vi "LHF.DB.Mongo.Client.GetCollectionsName.vi"(0 "LHF.DB.Mongo":refnum<class "LHF.DB.Mongo.lvclass">, 5 "error in (no error)":errorcluster) -> (14 "LHF.DB.Mongo":refnum<class "LHF.DB.Mongo.lvclass">, 15 "Collections":string[](array[string]))   [LabVIEW 2013, in "LHF.DB.Mongo.lvclass"]
uses:
  LHF.DB.Mongo.lvclass
  LHF.DB.Mongo.lvclass/LHF.DB.Mongo.ctl
  C:/Users/schim/Desktop/Projetos/LabVIEW-MongoDB/src/Driver/MongoDB.Driver.dll
  Driver/MongoDB.Driver.dll
  C:/Users/schim/Desktop/Projetos/LabVIEW-MongoDB/src/Driver/MongoDB.Bson.dll
  Driver/MongoDB.Bson.dll
panel:
  out "error out":errorcluster
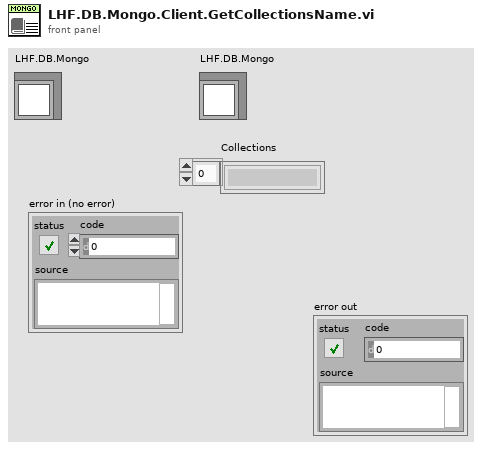
[diagram p1: front panel]
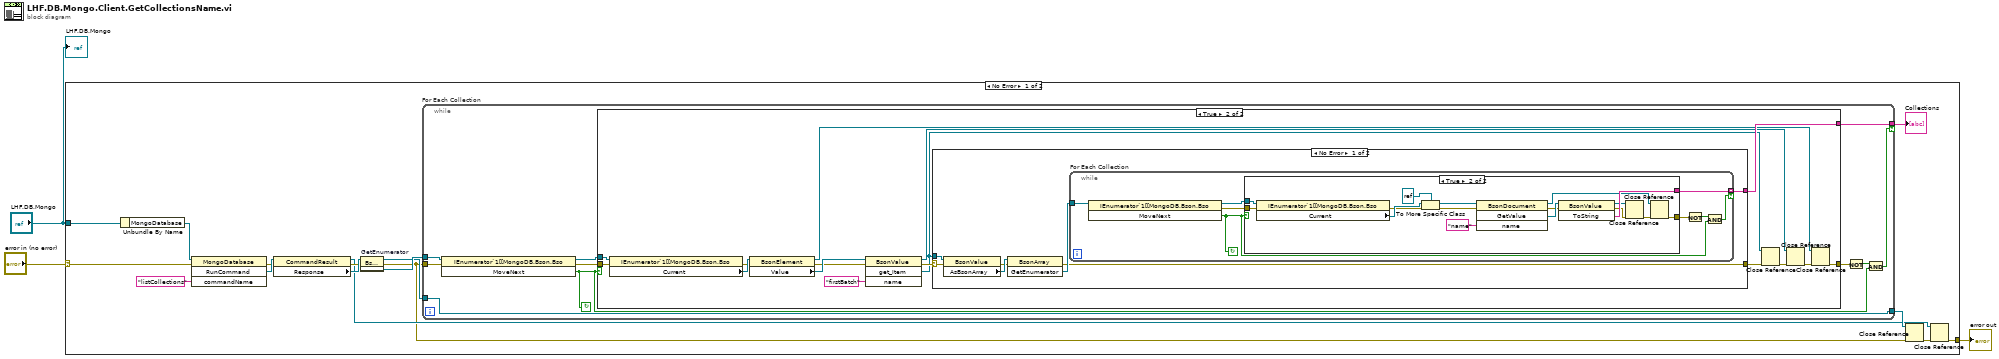
[diagram p0: block diagram]
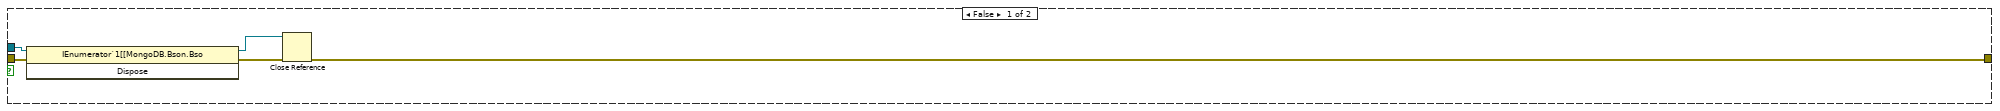
[diagram p2: hidden frame]
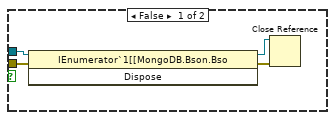
[diagram p3: hidden frame]
diagram:
  n1 = case shown="No Error" "error in (no error)" {
    selector: "error in (no error)" -> [w4 w87]
    tunnel: "LHF.DB.Mongo" -> [w15 _]
    tunnel: [w5 w87] -> w2
    frame No Error {
      n2 = Unbundle By Name(w15) -> ("MongoDatabase"=w14:refnum<k24>)
      n3 = invoke class="MongoDatabase" method="RunCommand"(reference=w14, error in=w4, "commandName"="listCollections") -> (error out=w10:errorcluster, "RunCommand"=w19:refnum<k24>)  [unwired: 1 in, 2 out]
      n4 = property class="CommandResult"(reference=w19, error in=w10) -> (reference out=w8:refnum<k24>, error out=w9:errorcluster, "Response"=w12:refnum<k24>)
      n5 = invoke on="GetEnumerator" class="BsonDocument" method="GetEnumerator"(reference=w12, error in=w9) -> (reference out=w17:refnum<k24>, error out=w6:errorcluster, "GetEnumerator"=w18:refnum<k24>)  [unwired: 1 in]
      n6 = while "For Each Collection" {
        tunnel: w18 -> [w29]
        tunnel: w17 -> [w26]
        tunnel: [w26] -> w16
        tunnel: [w25] -> w11 if=w21
        tunnel: w6 -> [w20]
        stop <- w22 continue-if-true
        n7 = invoke class="IEnumerator`1[[MongoDB.Bson.Bso" method="MoveNext"(reference=w29, error in=w20) -> (reference out=w28:refnum<k24>, error out=w27:errorcluster, "MoveNext"=w22:bool)  [unwired: 1 in]
        n8 = case shown="True" w22 {
          tunnel: w28 -> [w34 w50]
          tunnel: w27 -> [w31 w49]
          tunnel: [_ w42] -> w25
          tunnel: [w30 w35] -> w24
          frame False {
            n9 = invoke class="IEnumerator`1[[MongoDB.Bson.Bso" method="Dispose"(reference=w34, error in=w31) -> (reference out=w33:refnum<k24>, error out=w32:errorcluster)  [unwired: 1 in, 1 out]
            n10 = Close Reference(reference=w33, error in (no error)=w32) -> (error out=w30:errorcluster)
          }
          frame True {
            n11 = property class="IEnumerator`1[[MongoDB.Bson.Bso"(reference=w50, error in=w49) -> (error out=w44:errorcluster, "Current"=w48:refnum<k24>)  [unwired: 1 out]
            n12 = property class="BsonElement"(reference=w48, error in=w44) -> (reference out=w37:refnum<k24>, error out=w45:errorcluster, "Value"=w47:refnum<k24>)
            n13 = invoke class="BsonValue" method="get_Item"(reference=w47, error in=w45, "name"="firstBatch") -> (reference out=w39:refnum<k24>, error out=w43:errorcluster, "get_Item"=w41:refnum<k24>)  [unwired: 1 in, 1 out]
            n14 = case shown="No Error" w43 {
              selector: w43 -> [w53 w86]
              tunnel: w41 -> [w57 _]
              tunnel: [w52 _] -> w42
              tunnel: [w51 w86] -> w36
              frame No Error {
                n15 = property class="BsonValue"(reference=w57, error in=w53) -> (error out=w54:errorcluster, "AsBsonArray"=w56:refnum<k24>)  [unwired: 1 out]
                n16 = invoke class="BsonArray" method="GetEnumerator"(reference=w56, error in=w54) -> (error out=w51:errorcluster, "GetEnumerator"=w55:refnum<k24>)  [unwired: 1 in, 1 out]
                n17 = while "For Each Collection" {
                  tunnel: w55 -> [w63]
                  tunnel: [w62] -> w52 mode=indexing if=w58
                  stop <- w59 continue-if-true
                  n18 = invoke class="IEnumerator`1[[MongoDB.Bson.Bso" method="MoveNext"(reference=w63) -> (reference out=w65:refnum<k24>, error out=w64:errorcluster, "MoveNext"=w59:bool)  [unwired: 2 in]
                  n19 = case shown="True" w59 {
                    tunnel: w65 -> [w69 w85]
                    tunnel: w64 -> [w66 w84]
                    tunnel: [_ w78] -> w62
                    tunnel: [_ w70] -> w61
                    frame False {
                      n20 = invoke class="IEnumerator`1[[MongoDB.Bson.Bso" method="Dispose"(reference=w69, error in=w66) -> (reference out=w68:refnum<k24>, error out=w67:errorcluster)  [unwired: 1 in, 1 out]
                      n21 = Close Reference(reference=w68, error in (no error)=w67) -> ()  [unwired: 1 out]
                    }
                    frame True {
                      n22 = property class="IEnumerator`1[[MongoDB.Bson.Bso"(reference=w85, error in=w84) -> (error out=w77:errorcluster, "Current"=w83:refnum<k24>)  [unwired: 1 out]
                      n23 = To More Specific Class(target class=refnum<k24> refnum, reference=w83, error in=w77) -> (specific class reference=w81:refnum<k24>, error out=w76:errorcluster)
                      n24 = invoke class="BsonDocument" method="GetValue"(reference=w81, error in=w76, "name"="name") -> (reference out=w75:refnum<k24>, error out=w74:errorcluster, "GetValue"=w82:refnum<k24>)  [unwired: 1 in, 1 out]
                      n25 = invoke class="BsonValue" method="ToString"(reference=w82, error in=w74) -> (reference out=w72:refnum<k24>, error out=w73:errorcluster, "ToString"=w78:string)  [unwired: 1 in]
                      n26 = Close Reference(reference=w72, error in (no error)=w73) -> (error out=w71:errorcluster)
                      n27 = Close Reference(reference=w75, error in (no error)=w71) -> (error out=w70:errorcluster)
                    }
                  }
                  n28 = Not(x=w61) -> (.not. x?=w60:bool)
                  n29 = And(x=w60, y=w59) -> (x .and. y?=w58:bool)
                }
              }
              frame Error {
              }
            }
            n30 = Close Reference(reference=w41, error in (no error)=w36) -> (error out=w40:errorcluster)
            n31 = Close Reference(reference=w39, error in (no error)=w40) -> (error out=w38:errorcluster)
            n32 = Close Reference(reference=w37, error in (no error)=w38) -> (error out=w35:errorcluster)
          }
        }
        n33 = Not(x=w24) -> (.not. x?=w23:bool)
        n34 = And(x=w23, y=w22) -> (x .and. y?=w21:bool)
      }
      "Collections" <- w11
      n35 = Close Reference(reference=w16, error in (no error)=w6) -> (error out=w7:errorcluster)
      n36 = Close Reference(reference=w8, error in (no error)=w7) -> (error out=w5:errorcluster)
    }
    frame Error {
    }
  }
  "error out" <- w2
  "LHF.DB.Mongo" <- "LHF.DB.Mongo"
